vi "Telescope Move Focus.vi"(8 "error in (no error)":errorcluster, 10 "Focus Pos":dbl, 11 "Telescope Simulator in":refnum<class "Telescope Simulator.lvclass">) -> (0 "error out":errorcluster, 3 "Telescope Simulator out":refnum<class "Telescope Simulator.lvclass">)   [LabVIEW 2024, in "Telescope Simulator.lvclass"]
uses:
  Telescope Simulator.lvclass
  Telescope enum Status.ctl
  Telescope Simulator.lvclass/Telescope Simulator.ctl
  Telescope.lvclass
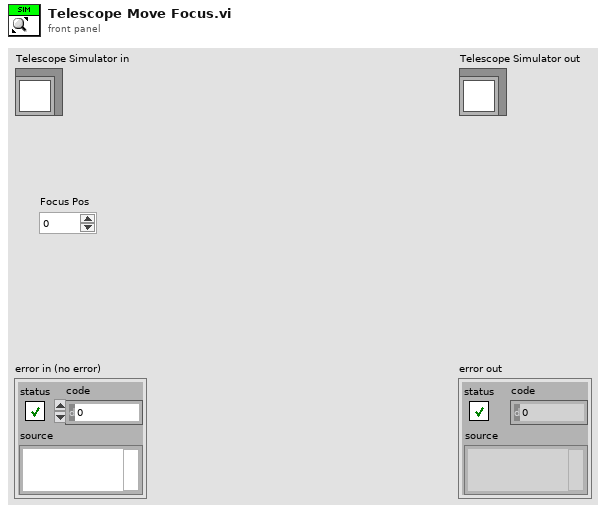
[diagram p1: front panel]
types:
  T1 = typedef "Telescope.lvclass/Telescope enum Status.ctl" = enum16{"Initializing", "Ready", "Moving", "Focusing", "Error"}
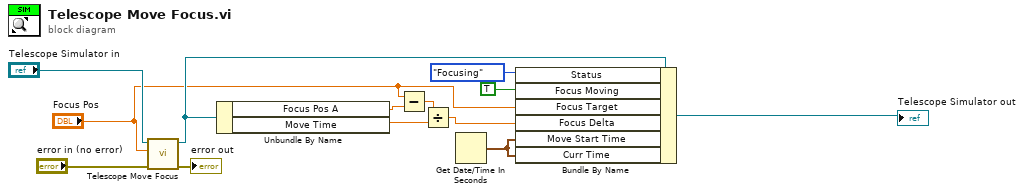
[diagram p0: block diagram]
diagram:
  n1 = call-parent "Telescope Move Focus.vi"("error in (no error)"="error in (no error)", "Focus Pos"="Focus Pos", "Telescope in"="Telescope Simulator in") -> ("error out"=→"error out":errorcluster, "Telescope out"=w5:refnum<class "Telescope Simulator.lvclass">)  [unwired: 7 in]
  n2 = Unbundle By Name(w5) -> ("Focus Pos A"=w4:dbl, "Move Time"=w10:dbl)
  n3 = Subtract(x="Focus Pos", y=w4) -> (x-y=w2:dbl)
  n4 = Divide(x=w2, y=w10) -> (x/y=w9:dbl)
  n5 = Get Date/Time In Seconds() -> (seconds since 1Jan1904=w7:timestamp)
  n6 = Bundle By Name(cluster=w5, "Status"=Telescope_enum_Status."Focusing" ("Telescope Status.Status"), "Focus Moving"=TRUE ("Focus.Focus Moving"), "Focus Target"="Focus Pos", "Focus Delta"=w9, "Move Start Time"=w7, "Curr Time"=w7) -> (→"Telescope Simulator out":refnum<class "Telescope Simulator.lvclass">)
